vi "Set Up auto (SubVI).vi"(5 "States in total":i32, 7 "Dots in total":i32) -> (4 "Dots of States":i32[][](array[numeric]))   [LabVIEW 2017]
panel:
  in  "Stop Button":bool=TRUE
  # "HERE YOU CAN ADD DOTS IN TASKS"
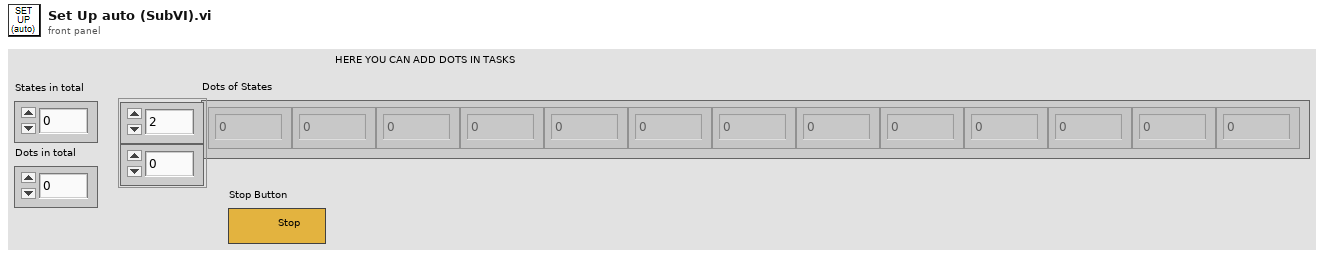
[diagram p1: front panel]
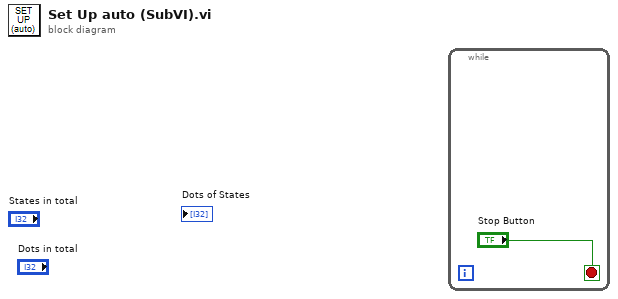
[diagram p0: block diagram]
diagram:
  n1 = while {
    stop <- "Stop Button" stop-if-true
  }
